vi "Save_USB_Config_File.vi"(0 "DAC Mode":i32, 1 "ADS Mode":i32, 2 "USB DAQ Vsup":dbl min=0.0 max=5.0, 3 "USB DAQ Vref":dbl min=0.0 max=5.0, 4 "USB DAQ Address":i32, 5 "App Path":path) -> ()   [LabVIEW 2011]
uses:
  <vilib>/Utility/config.llb/Write Key (Double).vi
  <vilib>/Utility/config.llb/Write Key (I32).vi
  <vilib>/Utility/config.llb/NI_LVConfig.lvlib
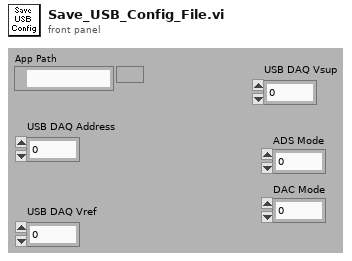
[diagram p1: front panel]
types:
  T1 = typedef "NI_LVConfig.lvlib/Config Data RefNum.ctl" = refnum<k1>
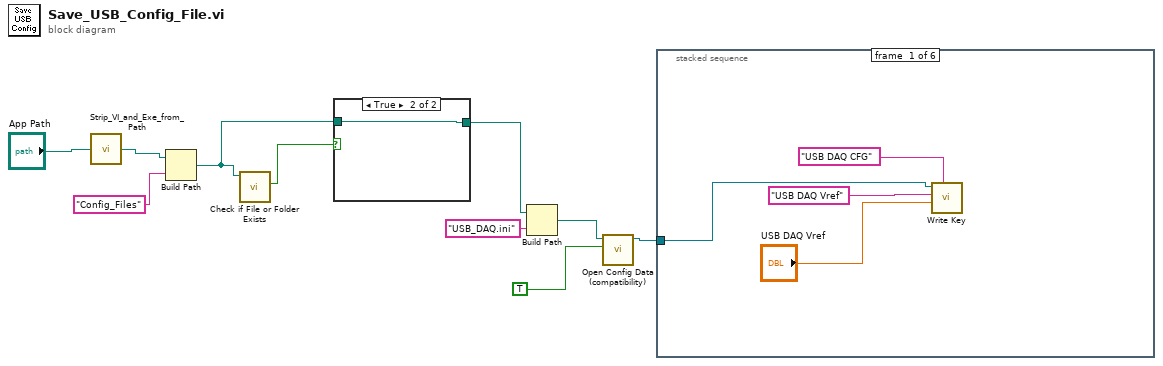
[diagram p0: block diagram]
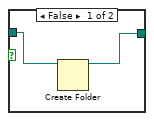
[diagram p2: hidden frame]
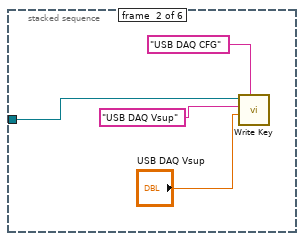
[diagram p3: hidden frame]
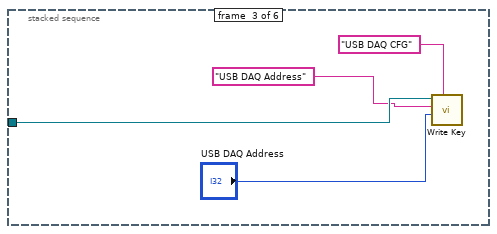
[diagram p4: hidden frame]
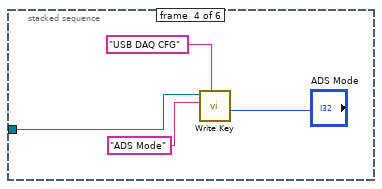
[diagram p5: hidden frame]
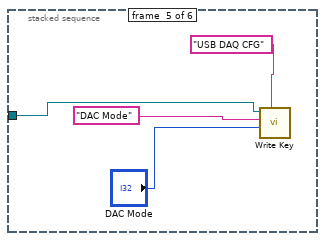
[diagram p6: hidden frame]
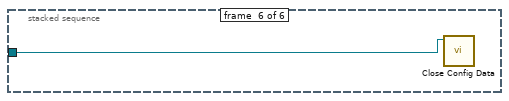
[diagram p7: hidden frame]
diagram:
  n1 = call "Strip_VI_and_Exe_from_Path.vi"("App Path"="App Path") -> ("App Path out"=w3:path)
  n2 = Build Path(base path=w3, name or relative path="Config_Files") -> (appended path=w2:path)
  n3 = call <vilib>:"Check if File or Folder Exists.vi"("path"=w2) -> ("file or folder exists?"=w5:bool)  [unwired: 8 in, 2 out]
  n4 = case shown="True" w5 {
    tunnel: w2 -> [w12 w13]
    tunnel: [w11 w13] -> w4
    frame False {
      n5 = Create Folder(path (use dialog)=w12) -> (created path=w11:path)  [unwired: 2 in, 2 out]
    }
    frame True {
    }
  }
  n6 = Build Path(base path=w4, name or relative path="USB_DAQ.ini") -> (appended path=w9:path)
  n7 = call <vilib>:"Open Config Data (compatibility).vi"("create file if necessary (T)"=TRUE ("create file if necessary? (T)"), "configuration file path"=w9) -> ("refnum"=w7:T1)  [unwired: 7 in, 2 out]
  n8 = stacked-sequence {
    tunnel: w7 -> [w14 w18 w25 w26 w30 w34]
    frame #0 {
      n9 = call-poly <vilib>:"Write Key.vi"("section"="USB DAQ CFG", "value"="USB DAQ Vref", "key"="USB DAQ Vref", "refnum"=w14) -> ()  [unwired: 5 in, 3 out]
    }
    frame #1 {
      n10 = call-poly <vilib>:"Write Key.vi"("section"="USB DAQ CFG", "value"="USB DAQ Vsup", "key"="USB DAQ Vsup" ("section"), "refnum"=w18) -> ()  [unwired: 5 in, 3 out]
    }
    frame #2 {
      n11 = call-poly <vilib>:"Write Key.vi"("section"="USB DAQ CFG", "value"="USB DAQ Address", "key"="USB DAQ Address" ("section"), "refnum"=w25) -> ()  [unwired: 5 in, 3 out]
    }
    frame #3 {
      n12 = call-poly <vilib>:"Write Key.vi"("section"="USB DAQ CFG", "value"="ADS Mode", "key"="ADS Mode" ("section"), "refnum"=w26) -> ()  [unwired: 5 in, 3 out]
    }
    frame #4 {
      n13 = call-poly <vilib>:"Write Key.vi"("section"="USB DAQ CFG", "value"="DAC Mode", "key"="DAC Mode" ("section"), "refnum"=w30) -> ()  [unwired: 5 in, 3 out]
    }
    frame #5 {
      n14 = call <vilib>:"Close Config Data.vi"("refnum"=w34) -> ()  [unwired: 9 in, 2 out]
    }
  }
